vi "Begin.vi"(8 "error in":errorcluster) -> (0 "error out":errorcluster)   [LabVIEW 2014]
doc: "Called before other user functions, this VI is expected to open initial I/O refnums, load in file data, and do all program initialization. Notice that the <B>error out</B> terminal is simply used for data flow. Wiring it to other structures or subVIs ensures that this VI runs first."
uses:
  <vilib>/Rock Robotics/SystemInterfaces/DIO/FPGA_DIOPWMChannel.ctl
  <vilib>/Rock Robotics/WPI/DriverStation/WPI_DriverStationRobotMode2.ctl
  <vilib>/Rock Robotics/SystemInterfaces/spilib/spi_bus.ctl
  <vilib>/Rock Robotics/SystemInterfaces/DIO/FPGA_DIOChannel.ctl
  <vilib>/Rock Robotics/WPI/Encoder/WPI_EncoderType.ctl
  <vilib>/Rock Robotics/WPI/Joystick/WPI_JoystickDeviceEnum.ctl
  <vilib>/Rock Robotics/SystemInterfaces/Typedef/FPGA_TypedefDigitalModule.ctl
  <vilib>/Rock Robotics/WPI/SafetyOutput/WPI_SafetyOutputConfigMenu.ctl
  <vilib>/Rock Robotics/WPI/Solenoid/WPI_SolenoidChannel.ctl
  <vilib>/Rock Robotics/WPI/RobotDrive/WPI_RobotDriveOpen2MotorWithTalon.vi
  Robot Global Data.vi
  <vilib>/Rock Robotics/Network Tables/SD Write String Array.vi
  <vilib>/Rock Robotics/WPI/Counter/WPI_CounterDigitalInputToDigitalSource.vi
  <vilib>/Rock Robotics/WPI/MotorControl/WPI_MotorControlOpen Talon.vi
  <vilib>/Rock Robotics/WPI/Solenoid/WPI_SolenoidOpenDouble.vi
  <vilib>/Rock Robotics/WPI/Accelerometer/InternalAccelerometer/WPI_AccelerometerInternalOpen.vi
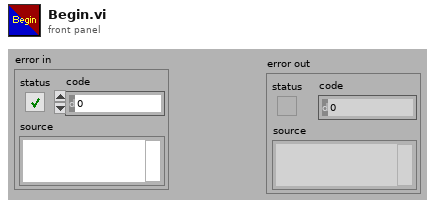
[diagram p1: front panel]
types:
  T1 = typedef "WPI_SolenoidChannel.ctl" = enum8{"Solenoid 0", "Solenoid 1", "Solenoid 2", "Solenoid 3", "Solenoid 4", "Solenoid 5", "Solenoid 6", "Solenoid 7", "Invalid"}
  T2 = typedef "WPI_SafetyOutputConfigMenu.ctl" = enum16{"Enable", "Disable"}
  T3 = typedef "FPGA_TypedefDigitalModule.ctl" = enum16{"Controller 1"}
  T4 = typedef "FPGA_DIOPWMChannel.ctl" = enum8{"PWM 0", "PWM 1", "PWM 2", "PWM 3", "PWM 4", "PWM 5", "PWM 6", "PWM 7", "PWM 8", "PWM 9", "PWM MXP 0", "PWM MXP 1", "PWM MXP 2", "PWM MXP 3", "PWM MXP 4", "PWM MXP 5", "PWM MXP 6", "PWM MXP 7", "PWM MXP 8", "PWM MXP 9", "Invalid"}
  T5 = typedef "WPI_JoystickDeviceEnum.ctl" = enum16{"USB 0", "USB 1", "USB 2", "USB 3", "USB 4", "USB 5"}
  T6 = typedef "WPI_EncoderType.ctl" = enum16{"1x", "2x", "4x"}
  T7 = typedef "FPGA_DIOChannel.ctl" = enum8{"DIO 0", "DIO 1", "DIO 2", "DIO 3", "DIO 4", "DIO 5", "DIO 6", "DIO 7", "DIO 8", "DIO 9", "DIO MXP 0", "DIO MXP 1", "DIO MXP 2", "DIO MXP 3", "DIO MXP 4", "DIO MXP 5", "DIO MXP 6", "DIO MXP 7", "DIO MXP 8", "DIO MXP 9", "DIO MXP 10", "DIO MXP 11", "DIO MXP 12", "DIO MXP 13", "DIO MXP 14", "DIO MXP 15", "Invalid"}
  T8 = typedef "spi_bus.ctl" = enum16{"SPI On-Board, CS0", "SPI On-Board, CS1", "SPI On-Board, CS2", "SPI On-Board, CS3", "SPI MXP", "Invalid"}
  T9 = typedef "WPI_DriverStationRobotMode2.ctl" = enum16{"Autonomous Disabled", "Autonomous Enabled", "Teleop Disabled", "Teleop Enabled", "Disconnected", "Finish", "Test Disabled", "Test Enabled", "Emergency Stopped"}
  T10 = typedef "WPI_JoystickDevRef.ctl" = cluster{"Device":T5}
  T11 = typedef "WPI_AccelerometerDevRef.ctl" = cluster{"DevStatus":errorcluster, "Controller":T12, "Scaling":T13, "Analog Channels":T14, "I2C Bus":T16, "SPI Bus":T8, "Accel Range":T17, "ADXL345 Axes":T18, "Handle":i32, "Device Address":u8, "Accel Type":enum16{"Analog", "ADXL345 I2C", "ADXL345 SPI", "Internal"}}
  T12 = typedef "FPGA_TypedefAnalogModule.ctl" = enum16{"Controller 1"}
  T13 = typedef "WPI_AccelerometerScaling.ctl" = cluster{"Gain (VoltsPerG)":dbl, "Center Voltage":dbl}
  T14 = typedef "WPI_AccelerometerAnalogChannels.ctl" = cluster{"X-Axis":T15, "Y-Axis":T15, "Z-Axis":T15}
  T15 = typedef "FPGA_AIChannel.ctl" = enum8{"AI 0", "AI 1", "AI 2", "AI 3", "AI MXP 0", "AI MXP 1", "AI MXP 2", "AI MXP 3", "Invalid"}
  T16 = typedef "i2c_bus.ctl" = enum16{"I2C On-Board", "I2C MXP", "Invalid"}
  T17 = typedef "ADXL345 Range.ctl" = u8
  T18 = typedef "WPI_AccelerometerADXL345 Axes.ctl" = cluster{"X-Axis":bool, "Y-Axis":bool, "Z-Axis":bool}
  T19 = typedef "WPI_RobotDriveDevRef.ctl" = cluster{"DevStatus":errorcluster, "Motors[]":T20[], "Square Inputs":bool, "Max Output":dbl}
  T20 = typedef "WPI_MotorControlDeviceRef.ctl" = cluster{"DeviceStatus":errorcluster, "Type":T21, "PWM":cluster{"Controller":T3, "PWM Channel":T4, "DeadBand":T22}, "CAN":cluster{"Device Number":u8, "Control Mode":T23, "Semaphore":T24, "Max Vout":dbl, "TalonSRX Control Mode":T25}, "Invert":bool, "TransformRef":T26, "InvTransformRef":T26}
  T21 = typedef "WPI_MotorControlType.ctl" = enum16{"PWM", "CAN", "CANTalonSRX"}
  T22 = typedef "WPI_PWMDeadband.ctl" = cluster{"Name":string, "maxPositivePwm":i32, "minPositivePwm":i32, "centerPwm":i32, "maxNegativePwm":i32, "minNegativePwm":i32, "angularRange":u16}
  T23 = typedef "WPI_CANJaguar_ControlMode.ctl" = enum8{"Percent VBus", "Current", "Speed", "Position", "Voltage"}
  T24 = typedef "Semaphore RefNum" = refnum<k1>
  T25 = typedef "WPI_CANTalonSRX_APIControlMode.ctl" = enum8{"Percent VBus", "Speed", "Position", "Slave", "Unchanged / Invalid"}
  T26 = typedef "WPI_PWMTransform_ConPane.ctl" = refnum<vi>
  T27 = typedef "WPI_SPIDevRef.ctl" = cluster{"DevStatus":errorcluster, "Handle":i32, "Controller":T3, "SPI Bus":T8}
  T28 = typedef "WPI_DigitalInputDevRef.ctl" = cluster{"DevStatus":errorcluster, "DIO Channel":T7, "Controller":T3}
  T29 = typedef "FPGA_CounterEncoderSourceConvertionLVSourceType.ctl" = cluster{"DevStatus":errorcluster, "AnalogTriggerMode?":bool, "DigitalMode":cluster{"Controller":T3, "DIO Channel":T30}, "AnalogTriggerMode":cluster{"AnalogTriggerIndex":T31, "OutputType":T32}}
  T30 = typedef "FPGA_DIODigitalSourceChannel.ctl" = enum8{"DIO 0", "DIO 1", "DIO 2", "DIO 3", "DIO 4", "DIO 5", "DIO 6", "DIO 7", "DIO 8", "DIO 9", "DIO MXP 0", "DIO MXP 1", "DIO MXP 2", "DIO MXP 3", "DIO MXP 4", "DIO MXP 5", "DIO MXP 6", "DIO MXP 7", "DIO MXP 8", "DIO MXP 9", "DIO MXP 10", "DIO MXP 11", "DIO MXP 12", "DIO MXP 13", "DIO MXP 14", "DIO MXP 15", "Disabled"}
  T31 = typedef "FPGA_AnalogTriggerIndex.ctl" = enum8{"Trig 0", "Trig 1", "Trig 2", "Trig 3", "Trig 4", "Trig 5", "Trig 6", "Trig 7", "Invalid"}
  T32 = typedef "FPGA_AnalogTriggerOutType.ctl" = enum16{"InWindow", "TriggerState", "Rising", "Falling"}
  T33 = typedef "WPI_EncoderDevRef.ctl" = cluster{"DevStatus":errorcluster, "EncoderIndex":T34, "CounterIndex":T35, "DistancePerCount":dbl, "Decoding Type":T6}
  T34 = typedef "FPGA_EncoderIdx.ctl" = enum8{"Enc 0", "Enc 1", "Enc 2", "Enc 3", "Enc 4", "Enc 5", "Enc 6", "Enc 7", "Invalid"}
  T35 = typedef "FPGA_CounterCtrSystemIndex.ctl" = enum8{"Ctr 0", "Ctr 1", "Ctr 2", "Ctr 3", "Ctr 4", "Ctr 5", "Ctr 6", "Ctr 7", "Invalid"}
  T36 = typedef "WPI_SolenoidDevRef.ctl" = cluster{"DevStatus":errorcluster, "Pneumatics Control Module":u8, "Forward Solenoid Channel":T1, "Reverse Solenoid Channel":T1}
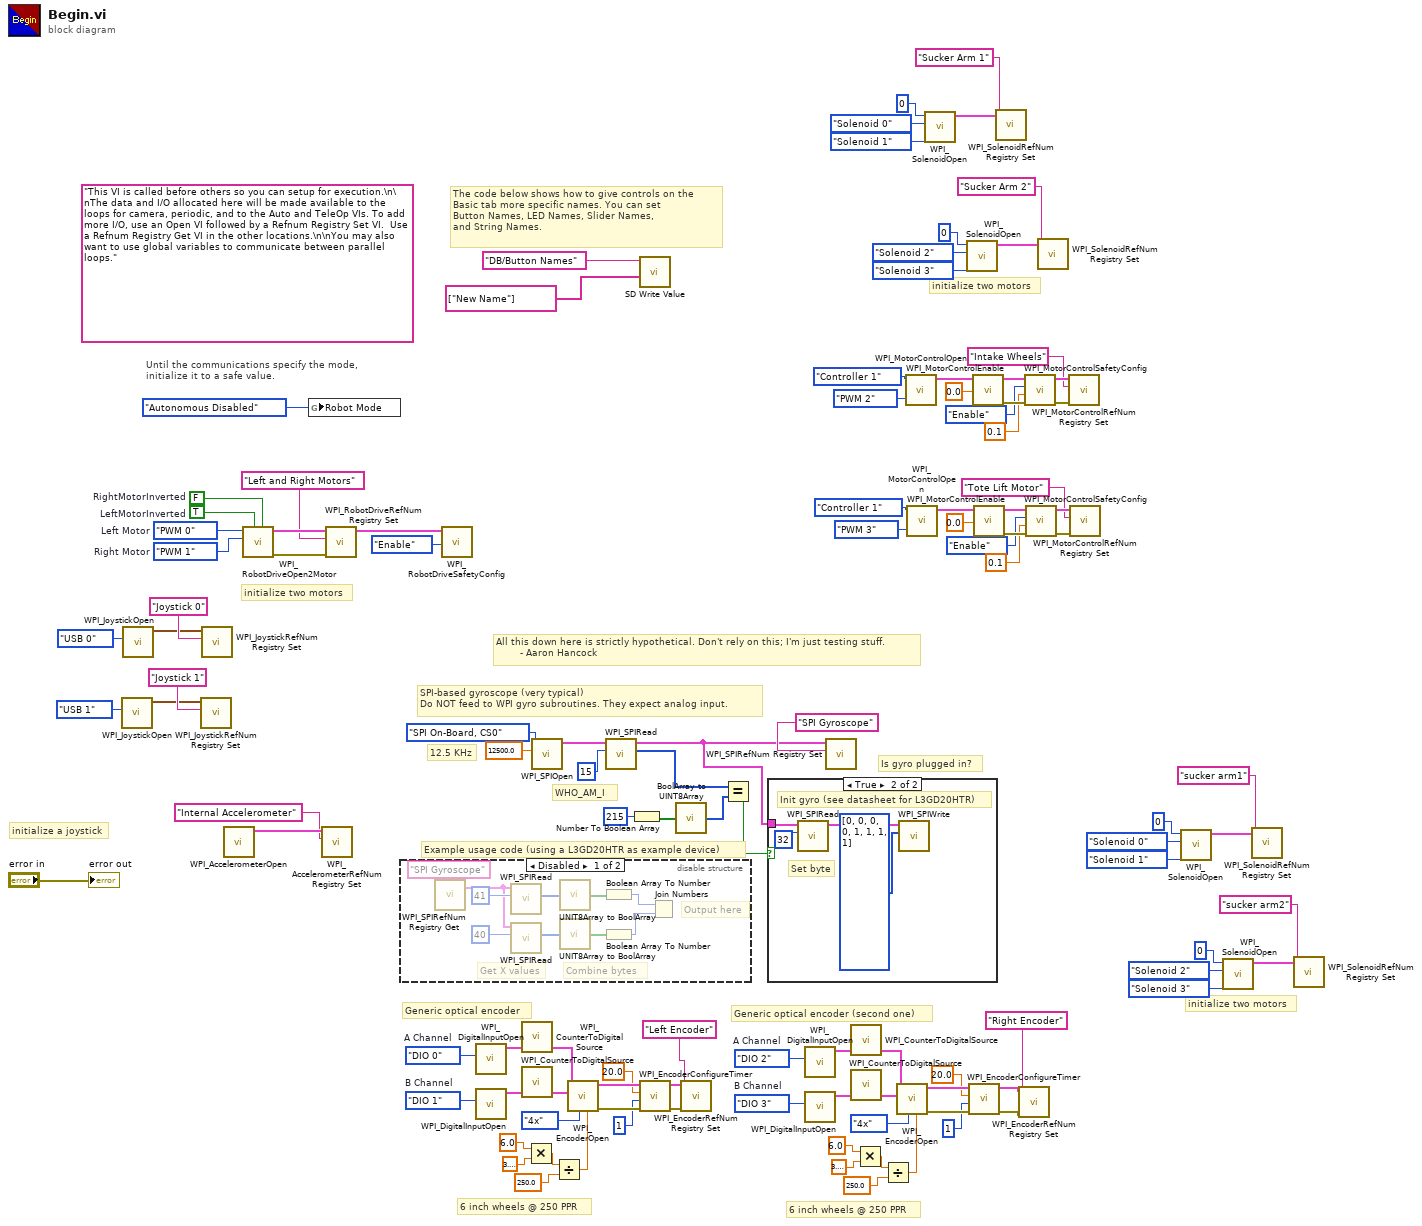
[diagram p0: block diagram]
diagram:
  w70 = FPGA_DIOChannel."DIO 3"  # B Channel
  w69 = FPGA_DIOChannel."DIO 2"  # A Channel
  w88 = FPGA_DIOChannel."DIO 1"  # B Channel
  w87 = FPGA_DIOChannel."DIO 0"  # A Channel
  (unwired) "This VI is called before others so you can setup for execution.\n\nThe data and I/O allocated here will be made available to the loops for camera, periodic, and to the Auto and TeleOp VIs. To add more I/O, use an Open VI followed by a Refnum Registry Set VI.  Use a Refnum Registry Get VI in the other locations.\n\nYou may also want to use global variables to communicate between parallel loops."
  w106 = FPGA_DIOPWMChannel."PWM 1"  # Right Motor
  w107 = FPGA_DIOPWMChannel."PWM 0"  # Left Motor
  w111 = TRUE  # LeftMotorInverted
  w112 = FALSE  # RightMotorInverted
  # "initialize two motors"
  # "initialize two motors"
  # "6 inch wheels @ 250 PPR"
  # "Generic optical encoder (second one)"
  # "6 inch wheels @ 250 PPR"
  # "Generic optical encoder"
  # "Is gyro plugged in?"
  # "WHO_AM_I"
  # "Example usage code (using a L3GD20HTR as example device)"
  # "12.5 KHz"
  # "SPI-based gyroscope (very typical)\nDo NOT feed to WPI gyro subroutines. They expect analog input."
  # "All this down here is strictly hypothetical. Don't rely on this; I'm just testing stuff.\n        - Aaron Hancock"
  # "The code below shows how to give controls on the\nBasic tab more specific names. You can set\nButton Names, LED Names, Slider Names,\nand String Names."
  # "initialize a joystick"
  # "Until the communications specify the mode,\ninitialize it to a safe value."
  # "initialize two motors"
  n1 = call <vilib>:"WPI_JoystickOpen.vi"("JoystickDevice"=WPI_JoystickDeviceEnum."USB 1") -> ("JoystickDevRef"=w44:T10)  [unwired: 10 in]
  n2 = call <vilib>:"WPI_JoystickOpen.vi"("JoystickDevice"=WPI_JoystickDeviceEnum."USB 0") -> ("JoystickDevRef"=w47:T10)  [unwired: 10 in]
  n3 = call <vilib>:"WPI_JoystickRefNum Registry Set.vi"("refnum name"="Joystick 1", "JoystickDevRef"=w44) -> ()  [unwired: 8 in, 2 out]
  n4 = call <vilib>:"WPI_JoystickRefNum Registry Set.vi"("refnum name"="Joystick 0", "JoystickDevRef"=w47) -> ()  [unwired: 8 in, 2 out]
  n5 = call-poly <vilib>:"WPI_AccelerometerOpen.vi"() -> ("AccelerometerDevRef"=w99:T11)  [unwired: 10 in, 1 out]
  n6 = call-poly <vilib>:"WPI_RobotDriveOpen2Motor.vi"("Right Motor Inverted"=w112, "Left Motor Inverted"=w111, "Right Motor"=w106, "Left Motor"=w107) -> ("error out"=w108:errorcluster, "RobotDriveDevRef"=w110:T19)  [unwired: 1 in, 5 out]
  n7 = global write "Robot Global Data.vi" "Robot Mode"(WPI_DriverStationRobotMode2."Autonomous Disabled" ("Robot Mode")) -> ()
  n8 = call <vilib>:"WPI_AccelerometerRefNum Registry Set.vi"("refnum name"="Internal Accelerometer", "AccelerometerDevRef"=w99) -> ()  [unwired: 8 in, 2 out]
  n9 = call <vilib>:"WPI_RobotDriveRefNum Registry Set.vi"("error in (no error)"=w108, "refnum name"="Left and Right Motors", "RobotDriveDevRef"=w110) -> ("RobotDriveDevRef"=w105:T19)  [unwired: 8 out]
  n10 = disable-structure shown="Disabled" {
    frame Disabled {
      # "Combine bytes"
      # "Output here"
      # "Get X values"
      n11 = call <vilib>:"WPI_SPIRefNum Registry Get.vi"("refnum name"="SPI Gyroscope") -> ("SPIDevRef"=w119:T27)  [unwired: 9 in, 1 out]
      n12 = call <vilib>:"WPI_SPIRead.vi"("Num to Read"=41, "SPIDevRef"=w119) -> ("Received Data"=w118:u8[])  [unwired: 7 in, 2 out]
      n13 = call <vilib>:"WPI_SPIRead.vi"("Num to Read"=40, "SPIDevRef"=w119) -> ("Received Data"=w117:u8[])  [unwired: 7 in, 2 out]
      n14 = call "UNIT8Array to BoolArray.vi"("Input Array (UINT_8)"=w118) -> ("Output Array (Bool)"=w116:bool[])
      n15 = call "UNIT8Array to BoolArray.vi"("Input Array (UINT_8)"=w117) -> ("Output Array (Bool)"=w115:bool[])
      n16 = Boolean Array To Number(Boolean array=w116) -> (number=w114:u32)
      n17 = Boolean Array To Number(Boolean array=w115) -> (number=w113:u32)
      n18 = Join Numbers(hi=w114, lo=w113) -> ()  [unwired: 1 out]
    }
    frame Enabled {
    }
  }
  n19 = call <vilib>:"WPI_RobotDriveSafetyConfig.vi"("mode"=WPI_SafetyOutputConfigMenu."Enable", "RobotDriveDevRef"=w105) -> ()  [unwired: 8 in, 2 out]
  n20 = call <vilib>:"WPI_DigitalInputOpen.vi"("DIO Channel"=w87) -> ("DigitalInputDevRef"=w84:T28)  [unwired: 2 in, 8 out]
  n21 = call <vilib>:"WPI_DigitalInputOpen.vi"("DIO Channel"=w88) -> ("DigitalInputDevRef"=w85:T28)  [unwired: 2 in, 8 out]
  n22 = call-poly <vilib>:"WPI_CounterToDigitalSource.vi"("DigitalInputDevRef"=w84) -> ("Digital Source"=w83:T29)  [unwired: 6 out]
  n23 = call-poly <vilib>:"WPI_CounterToDigitalSource.vi"("DigitalInputDevRef"=w85) -> ("Digital Source"=w86:T29)  [unwired: 6 out]
  n24 = Multiply(x=6.0 ("DistancePerCount"), y=3.141592653589793) -> (x*y=w75:dbl)
  n25 = call <vilib>:"WPI_SPIOpen.vi"("Clock Rate (Hz)"=12500.0, "SPI Bus"=spi_bus."SPI On-Board, CS0") -> ("SPIDevRef"=w52:T27)  [unwired: 8 in, 1 out]
  n26 = Divide(x=w75, y=250.0 ("DistancePerCount")) -> (x/y=w73:dbl)
  n27 = call <vilib>:"WPI_EncoderOpen.vi"("DistancePerCount"=w73, "Decoding Type"=WPI_EncoderType."4x", "BSource"=w86, "ASource"=w83) -> ("error out"=w79:errorcluster, "EncoderDevRef"=w78:T33)  [unwired: 4 in, 2 out]
  n28 = call <vilib>:"WPI_SPIRead.vi"("Num to Read"=15, "SPIDevRef"=w52) -> ("Received Data"=w90:u8[], "SPIDevRef"=w53:T27)  [unwired: 7 in, 1 out]
  n29 = Number To Boolean Array(number=u32 215) -> (Boolean array=w92:bool[])
  n30 = call-poly <vilib>:"SD Write Value.vi"("String Array"=string[] ["New Name"], "Name"="DB/Button Names") -> ()  [unwired: 8 in, 2 out]
  n31 = call <vilib>:"WPI_EncoderConfigureTimer.vi"("error in (no error)"=w79, "Number Samples to Average"=u8 1, "Minimum Rate"=20.0, "EncoderDevRef"=w78) -> ("error out"=w72:errorcluster, "EncoderDevRef"=w71:T33)  [unwired: 6 in]
  n32 = call "BoolArray to UINT8Array.vi"("Input Array (Bool)"=w92) -> ("Output Array (UINT_8)"=w91:u8[])
  n33 = call <vilib>:"WPI_EncoderRefNum Registry Set.vi"("error in (no error)"=w72, "refnum name"="Left Encoder", "EncoderDevRef"=w71) -> ()  [unwired: 7 in, 2 out]
  n34 = Equal?(x=w90, y=w91) -> (x = y?=w89:bool)
  n35 = case shown="True" w89 {
    tunnel: w53 -> [_ w125]
    frame False {
    }
    frame True {
      # "Set byte"
      # "Init gyro (see datasheet for L3GD20HTR)"
      n36 = call <vilib>:"WPI_SPIRead.vi"("Num to Read"=32, "SPIDevRef"=w125) -> ("SPIDevRef"=w124:T27)  [unwired: 7 in, 2 out]
      n37 = call <vilib>:"WPI_SPIWrite.vi"("Data To Send"=u8[] [0, 0, 0, 0, 1, 1, 1, 1], "SPIDevRef"=w124) -> ()  [unwired: 7 in, 3 out]
    }
  }
  n38 = call <vilib>:"WPI_DigitalInputOpen.vi"("DIO Channel"=w69) -> ("DigitalInputDevRef"=w66:T28)  [unwired: 2 in, 8 out]
  n39 = call <vilib>:"WPI_DigitalInputOpen.vi"("DIO Channel"=w70) -> ("DigitalInputDevRef"=w67:T28)  [unwired: 2 in, 8 out]
  n40 = call <vilib>:"WPI_SPIRefNum Registry Set.vi"("refnum name"="SPI Gyroscope", "SPIDevRef"=w53) -> ()  [unwired: 8 in, 2 out]
  n41 = call-poly <vilib>:"WPI_CounterToDigitalSource.vi"("DigitalInputDevRef"=w66) -> ("Digital Source"=w65:T29)  [unwired: 6 out]
  n42 = call-poly <vilib>:"WPI_CounterToDigitalSource.vi"("DigitalInputDevRef"=w67) -> ("Digital Source"=w68:T29)  [unwired: 6 out]
  n43 = Multiply(x=6.0 ("DistancePerCount"), y=3.141592653589793) -> (x*y=w57:dbl)
  n44 = Divide(x=w57, y=250.0 ("DistancePerCount")) -> (x/y=w55:dbl)
  n45 = call <vilib>:"WPI_EncoderOpen.vi"("DistancePerCount"=w55, "Decoding Type"=WPI_EncoderType."4x", "BSource"=w68, "ASource"=w65) -> ("error out"=w61:errorcluster, "EncoderDevRef"=w60:T33)  [unwired: 4 in, 2 out]
  n46 = call-poly <vilib>:"WPI_MotorControlOpen.vi"("PWM Channel"=FPGA_DIOPWMChannel."PWM 2", "Controller"=FPGA_TypedefDigitalModule."Controller 1") -> ("MotorControlDeviceRef"=w40:T20)  [unwired: 8 in, 1 out]
  n47 = call-poly <vilib>:"WPI_MotorControlOpen.vi"("PWM Channel"=FPGA_DIOPWMChannel."PWM 3", "Controller"=FPGA_TypedefDigitalModule."Controller 1") -> ("MotorControlDeviceRef"=w29:T20)  [unwired: 8 in, 1 out]
  n48 = call-poly <vilib>:"WPI_SolenoidOpen.vi"("Reverse Solenoid Channel"=WPI_SolenoidChannel."Solenoid 1", "Forward Solenoid Channel"=WPI_SolenoidChannel."Solenoid 0", "Pneumatics Control Module (0)"=u8 0) -> ("SolenoidDevRef"=w7:T36)  [unwired: 7 in, 1 out]
  n49 = call-poly <vilib>:"WPI_SolenoidOpen.vi"("Reverse Solenoid Channel"=WPI_SolenoidChannel."Solenoid 3", "Forward Solenoid Channel"=WPI_SolenoidChannel."Solenoid 2", "Pneumatics Control Module (0)"=u8 0) -> ("SolenoidDevRef"=w2:T36)  [unwired: 7 in, 1 out]
  n50 = call <vilib>:"WPI_EncoderConfigureTimer.vi"("error in (no error)"=w61, "Number Samples to Average"=u8 1, "Minimum Rate"=20.0, "EncoderDevRef"=w60) -> ("error out"=w54:errorcluster, "EncoderDevRef"=w51:T33)  [unwired: 6 in]
  n51 = call <vilib>:"WPI_MotorControlEnable.vi"("Encoder Initial Position"=0.0, "CAN Jaguar Ref"=w40) -> ("error out"=w38:errorcluster, "CAN Jaguar Ref Out"=w37:T20)  [unwired: 8 in]
  n52 = call <vilib>:"WPI_MotorControlEnable.vi"("Encoder Initial Position"=0.0, "CAN Jaguar Ref"=w29) -> ("error out"=w27:errorcluster, "CAN Jaguar Ref Out"=w26:T20)  [unwired: 8 in]
  n53 = call <vilib>:"WPI_SolenoidRefNum Registry Set.vi"("refnum name"="Sucker Arm 1", "SolenoidDevRef"=w7) -> ()  [unwired: 8 in, 2 out]
  n54 = call <vilib>:"WPI_EncoderRefNum Registry Set.vi"("error in (no error)"=w54, "refnum name"="Right Encoder", "EncoderDevRef"=w51) -> ()  [unwired: 7 in, 2 out]
  n55 = call <vilib>:"WPI_MotorControlSafetyConfig.vi"("error in (no error)"=w38, "timeout (s)"=0.1, "mode"=WPI_SafetyOutputConfigMenu."Enable", "MotorControlDevRef"=w37) -> ("error out"=w34:errorcluster, "MotorControlDevRef"=w33:T20)  [unwired: 6 in]
  n56 = call <vilib>:"WPI_MotorControlSafetyConfig.vi"("error in (no error)"=w27, "timeout (s)"=0.1, "mode"=WPI_SafetyOutputConfigMenu."Enable", "MotorControlDevRef"=w26) -> ("error out"=w23:errorcluster, "MotorControlDevRef"=w22:T20)  [unwired: 6 in]
  n57 = call <vilib>:"WPI_SolenoidRefNum Registry Set.vi"("refnum name"="Sucker Arm 2", "SolenoidDevRef"=w2) -> ()  [unwired: 8 in, 2 out]
  n58 = call <vilib>:"WPI_MotorControlRefNum Registry Set.vi"("error in (no error)"=w34, "refnum name"="Intake Wheels", "MotorControlDevRef"=w33) -> ()  [unwired: 7 in, 2 out]
  n59 = call <vilib>:"WPI_MotorControlRefNum Registry Set.vi"("error in (no error)"=w23, "refnum name"="Tote Lift Motor", "MotorControlDevRef"=w22) -> ()  [unwired: 7 in, 2 out]
  n60 = call-poly <vilib>:"WPI_SolenoidOpen.vi"("Reverse Solenoid Channel"=WPI_SolenoidChannel."Solenoid 1", "Forward Solenoid Channel"=WPI_SolenoidChannel."Solenoid 0", "Pneumatics Control Module (0)"=u8 0) -> ("SolenoidDevRef"=w17:T36)  [unwired: 7 in, 1 out]
  n61 = call-poly <vilib>:"WPI_SolenoidOpen.vi"("Reverse Solenoid Channel"=WPI_SolenoidChannel."Solenoid 3", "Forward Solenoid Channel"=WPI_SolenoidChannel."Solenoid 2", "Pneumatics Control Module (0)"=u8 0) -> ("SolenoidDevRef"=w12:T36)  [unwired: 7 in, 1 out]
  n62 = call <vilib>:"WPI_SolenoidRefNum Registry Set.vi"("refnum name"="sucker arm1", "SolenoidDevRef"=w17) -> ()  [unwired: 8 in, 2 out]
  n63 = call <vilib>:"WPI_SolenoidRefNum Registry Set.vi"("refnum name"="sucker arm2", "SolenoidDevRef"=w12) -> ()  [unwired: 8 in, 2 out]
  "error out" <- "error in"
